vi "Input Voltage and Hysteresis Calibration.vi"(5 "Diagnostic Parameter (0: Off)":i32(ring) items=["Off", "Once"], 7 "Type (0: Calibration of Hysteresis Compensation)":i32(ring) items=["Calibration of Hysteresis Compensation", "DC Voltage Calibration", "Input Comparator Hysteresis Calibration"], 8 "error in (no error)":errorcluster, 9 "Value (0)":dbl, 10 "Channel (0: A)":i32(ring) items=["A", "B"], 11 "VISA resource name":refnum<visa-resource-name>) -> (0 "error out":errorcluster, 3 "VISA resource name out":refnum<visa-resource-name>)   [LabVIEW 2019, in "Pendulum CNT90.lvlib"]
doc: "Performs hysteresis compensation of the input comparators. No external input signal is allowed during the process. Or calibrates a DC voltage within the range from -50 V to +50 V if the corresponding voltage from a voltage reference source is applied to the input that is addressed in the command. Or measures and saves the hysteresis levels of the input comparator."
uses:
  Pendulum CNT90.lvlib
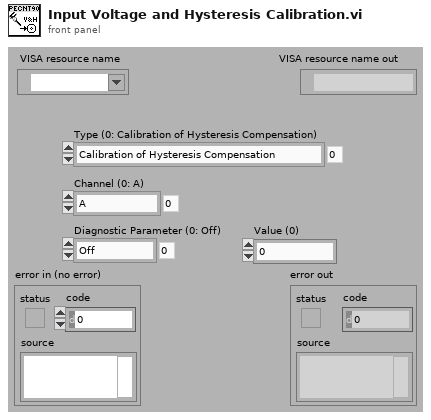
[diagram p1: front panel]
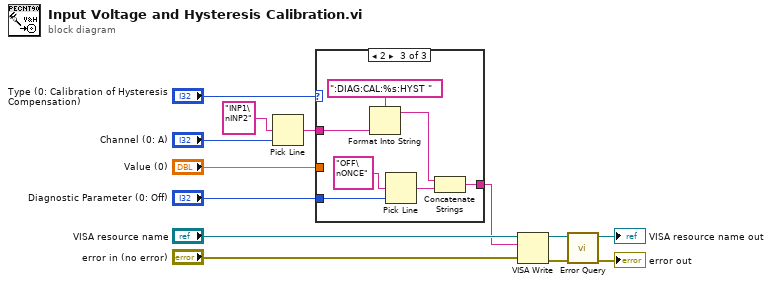
[diagram p0: block diagram]
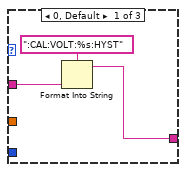
[diagram p2: hidden frame]
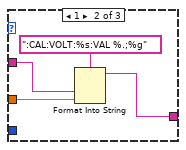
[diagram p3: hidden frame]
diagram:
  n1 = Pick Line(multi-line string="INP1\nINP2", line index="Channel (0: A)") -> (output string=w4:string)  [unwired: 1 in]
  n2 = case shown="2" "Type (0: Calibration of Hysteresis Compensation)" {
    tunnel: w4 -> [w16 w19 w22]
    tunnel: "Value (0)" -> [_ w18 _]
    tunnel: "Diagnostic Parameter (0: Off)" -> [_ _ w27]
    tunnel: [w14 w17 w24] -> w1
    frame 0, Default {
      n3 = Format Into String(format string=":CAL:VOLT:%s:HYST", w16) -> (resulting string=w14:string)  [unwired: 2 in, 1 out]
    }
    frame 1 {
      n4 = Format Into String(format string=":CAL:VOLT:%s:VAL %.;%g", w19, w18) -> (resulting string=w17:string)  [unwired: 2 in, 1 out]
    }
    frame 2 {
      n5 = Format Into String(format string=":DIAG:CAL:%s:HYST ", w22) -> (resulting string=w21:string)  [unwired: 2 in, 1 out]
      n6 = Pick Line(multi-line string="OFF\nONCE", line index=w27) -> (output string=w25:string)  [unwired: 1 in]
      n7 = Concatenate Strings(w21, w25) -> (w24:string)
    }
  }
  n8 = VISA Write(VISA resource name="VISA resource name", write buffer=w1, error in (no error)="error in (no error)") -> (VISA resource name out=w11:refnum<visa-resource-name>, error out=w8:errorcluster)  [unwired: 1 out]
  n9 = call "Error Query.vi"("error in (no error)"=w8, "VISA resource name"=w11) -> ("error out"=→"error out":errorcluster, "VISA resource name out"=→"VISA resource name out":refnum<visa-resource-name>)  [unwired: 6 in, 2 out]
